vi "Config Interactive Ctrl logic.vi"(6 "Test Val Ref":refnum<vi>, 7 "Data":variant, 8 "error in (no error)":errorcluster, 9 "Commit Ref":refnum<vi>, 10 "Next Ref":refnum<vi>, 11 "Start/Prev Ref":refnum<vi>) -> (0 "error out":errorcluster)   [LabVIEW 2018, in "Testing UI 1.lvlib"]
uses:
  Testing UI 1.lvlib
  Public Controls/Config Interactive Buttons.ctl
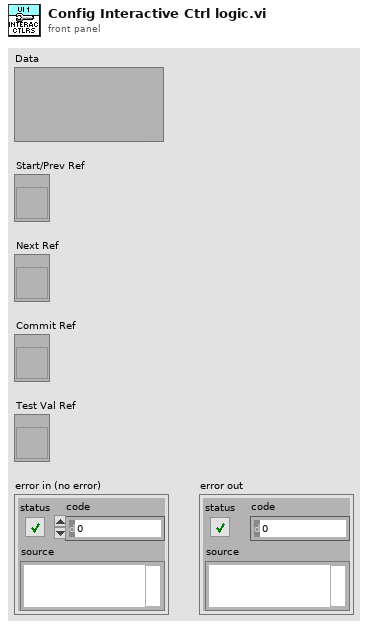
[diagram p1: front panel]
types:
  T1 = enum8{"Enabled", "Disabled", "Disabled and Grayed Out"}
  T2 = typedef "Testing UI 1.lvlib/Config Interactive Buttons.ctl" = cluster{"Start/Prev (en/dis)":bool, "Next (en/dis)":bool, "Commit(en/dis)":bool, "Test Value (en/dis)":bool, "Start/Prev (Cap)":string, "Next (Cap)":string, "Commit (Cap)":string, " Test Val (Cap)":string}
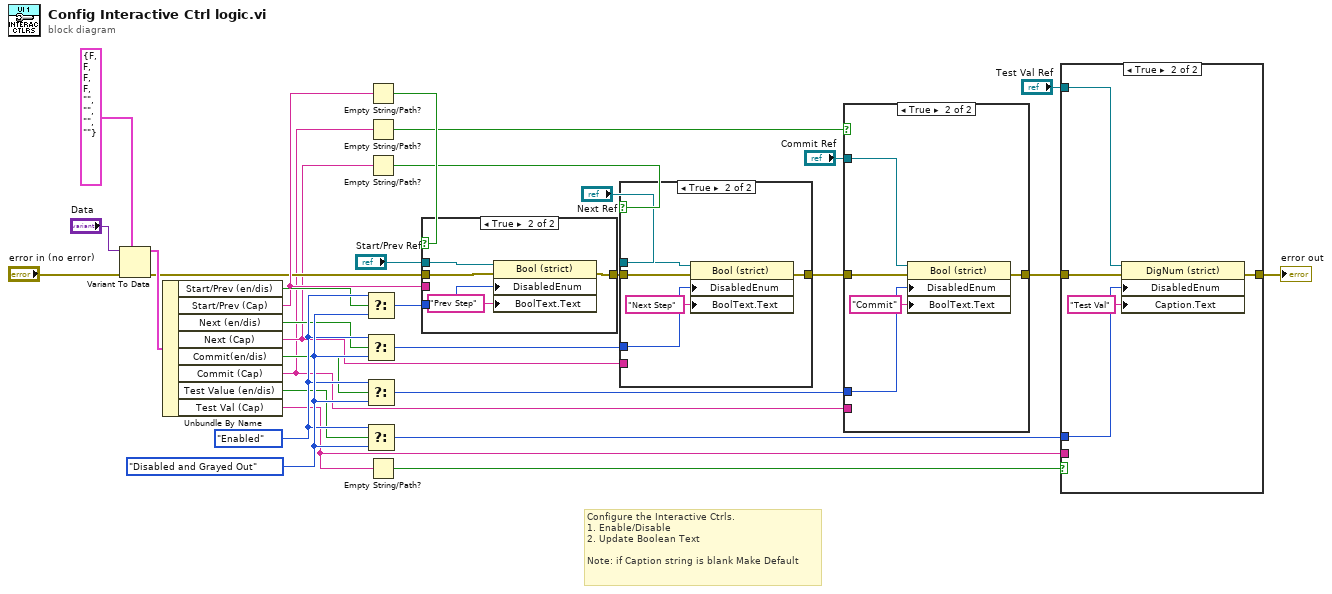
[diagram p0: block diagram]
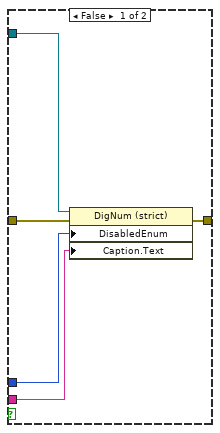
[diagram p2: hidden frame]
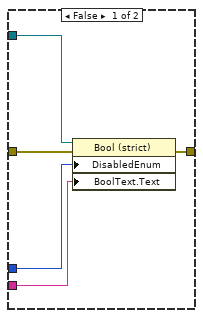
[diagram p3: hidden frame]
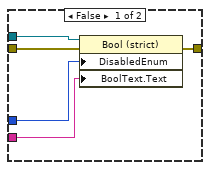
[diagram p4: hidden frame]
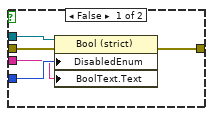
[diagram p5: hidden frame]
diagram:
  w31 = T1."Disabled and Grayed Out" ("Disabled")
  w30 = T1."Enabled" ("Disabled")
  # "Configure the Interactive Ctrls.\n1. Enable/Disable\n2. Update Boolean Text\n\nNote: if Caption string is blank Make Default"
  n1 = Variant To Data(error in="error in (no error)", type=T2 {"Start/Prev (en/dis)"=FALSE, "Next (en/dis)"=FALSE, "Commit(en/dis)"=FALSE, "Test Value (en/dis)"=FALSE, "Start/Prev (Cap)"="", "Next (Cap)"="", "Commit (Cap)"="", " Test Val (Cap)"=""} ("Config Interactive Buttons"), Variant="Data") -> (data=w25:T2, error out=w17:errorcluster)
  n2 = Unbundle By Name(w25) -> ("Start/Prev (en/dis)"=w26:bool, "Start/Prev (Cap)"=w18:string, "Next (en/dis)"=w27:bool, "Next (Cap)"=w14:string, "Commit(en/dis)"=w28:bool, "Commit (Cap)"=w7:string, "Test Value (en/dis)"=w29:bool, "Test Val (Cap)"=w2:string)
  n3 = Select(t=w30, s=w26, f=w31) -> (s? t:f=w19:T1)
  n4 = Select(t=w30, s=w27, f=w31) -> (s? t:f=w12:T1)
  n5 = Select(t=w30, s=w28, f=w31) -> (s? t:f=w10:T1)
  n6 = Select(t=w30, s=w29, f=w31) -> (s? t:f=w4:T1)
  n7 = Empty String/Path?(string/path=w18) -> (empty?=w21:bool)
  n8 = Empty String/Path?(string/path=w7) -> (empty?=w8:bool)
  n9 = Empty String/Path?(string/path=w14) -> (empty?=w15:bool)
  n10 = Empty String/Path?(string/path=w2) -> (empty?=w1:bool)
  n11 = case shown="True" w21 {
    tunnel: "Start/Prev Ref" -> [w34 w41]
    tunnel: w19 -> [w36 w40]
    tunnel: w18 -> [w35 _]
    tunnel: w17 -> [w33 w39]
    tunnel: [w32 w38] -> w16
    frame False {
      n12 = property on="Property Node" class="Bool (strict)"(reference=w34, error in=w33, "DisabledEnum"=w36, "BoolText.Text"=w35) -> (error out=w32:errorcluster)  [unwired: 1 out]
    }
    frame True {
      n13 = property on="Property Node" class="Bool (strict)"(reference=w41, error in=w39, "DisabledEnum"=w40, "BoolText.Text"="Prev Step" ("Boolean Text.Text")) -> (error out=w38:errorcluster)  [unwired: 1 out]
    }
  }
  n14 = case shown="True" w15 {
    tunnel: w16 -> [w46 w51]
    tunnel: w14 -> [w45 _]
    tunnel: "Next Ref" -> [w44 w50]
    tunnel: w12 -> [w43 w49]
    tunnel: [w42 w48] -> w9
    frame False {
      n15 = property on="Property Node" class="Bool (strict)"(reference=w44, error in=w46, "DisabledEnum"=w43, "BoolText.Text"=w45) -> (error out=w42:errorcluster)  [unwired: 1 out]
    }
    frame True {
      n16 = property on="Property Node" class="Bool (strict)"(reference=w50, error in=w51, "DisabledEnum"=w49, "BoolText.Text"="Next Step" ("Boolean Text.Text")) -> (error out=w48:errorcluster)  [unwired: 1 out]
    }
  }
  n17 = case shown="True" w8 {
    tunnel: w9 -> [w56 w61]
    tunnel: w7 -> [w55 _]
    tunnel: "Commit Ref" -> [w54 w60]
    tunnel: w10 -> [w53 w59]
    tunnel: [w52 w58] -> w5
    frame False {
      n18 = property on="Property Node" class="Bool (strict)"(reference=w54, error in=w56, "DisabledEnum"=w53, "BoolText.Text"=w55) -> (error out=w52:errorcluster)  [unwired: 1 out]
    }
    frame True {
      n19 = property on="Property Node" class="Bool (strict)"(reference=w60, error in=w61, "DisabledEnum"=w59, "BoolText.Text"="Commit" ("Boolean Text.Text")) -> (error out=w58:errorcluster)  [unwired: 1 out]
    }
  }
  n20 = case shown="True" w1 {
    tunnel: w5 -> [w66 w71]
    tunnel: "Test Val Ref" -> [w65 w70]
    tunnel: w4 -> [w64 w69]
    tunnel: w2 -> [w63 _]
    tunnel: [w62 w68] -> w3
    frame False {
      n21 = property on="Property Node" class="DigNum (strict)"(reference=w65, error in=w66, "DisabledEnum"=w64, "Caption.Text"=w63) -> (error out=w62:errorcluster)  [unwired: 1 out]
    }
    frame True {
      n22 = property on="Property Node" class="DigNum (strict)"(reference=w70, error in=w71, "DisabledEnum"=w69, "Caption.Text"="Test Val") -> (error out=w68:errorcluster)  [unwired: 1 out]
    }
  }
  "error out" <- w3
